vi "ADCP_get_data_packet_list.vi"(8 "error in (no error)":errorcluster, 9 "Node name":string, 10 "Node ID":i32=-1, 11 "ADCP In":refnum<class "ADCP.lvclass">) -> (0 "error out":errorcluster, 1 "Data packets names":string[](array[string]), 2 "Data packets":T2(array[cluster]), 3 "ADCP Out":refnum<class "ADCP.lvclass">)   [LabVIEW 2017, in "ADCP.lvclass"]
uses:
  ADCP.lvclass
  ADCP_Data_Packet_Transmit_Mode.ctl
  ADCP.lvclass/ADCP.ctl
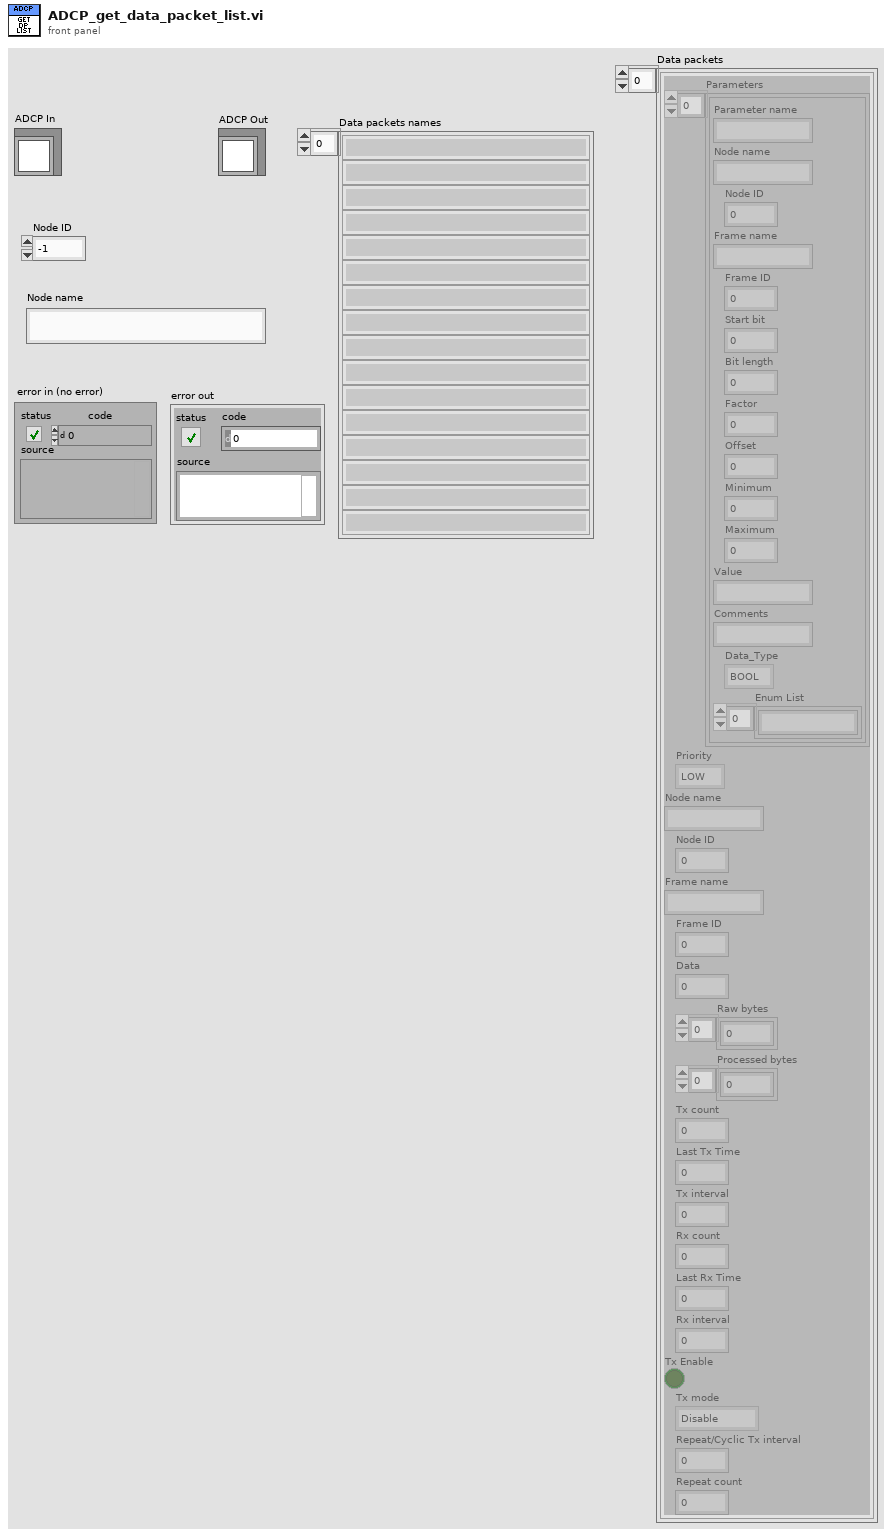
[diagram p1: front panel]
types:
  T1 = typedef "ADCP.lvclass/ADCP_Data_Packet_Transmit_Mode.ctl" = enum16{"Disable", "Single", "Cyclic", "Repeat"}
  T2 = cluster{"Parameters":cluster{"Parameter name":string, "Node name":string, "Node ID":u8, "Frame name":string, "Frame ID":u8, "Start bit":u32, "Bit length":u32, "Factor":dbl, "Offset":dbl, "Minimum":dbl, "Maximum":dbl, "Value":string, "Comments":string, "Data_Type":enum16{"BOOL", "UNSIGNED", "SIGNED", "FLOAT32", "ENUM"}, "Enum List":string[]}[], "Priority":enum16{"LOW", "HIGH"}, "Node name":string, "Node ID":u8, "Frame name":string, "Frame ID":u8, "Data":u32, "Raw bytes":u8[], "Processed bytes":u8[], "Tx count":i32, "Last Tx Time":u32, "Tx interval":u32, "Rx count":i32, "Last Rx Time":u32, "Rx interval":u32, "Tx Enable":bool, "Tx mode":T1, "Repeat/Cyclic Tx interval":u32, "Repeat count":u16}[]
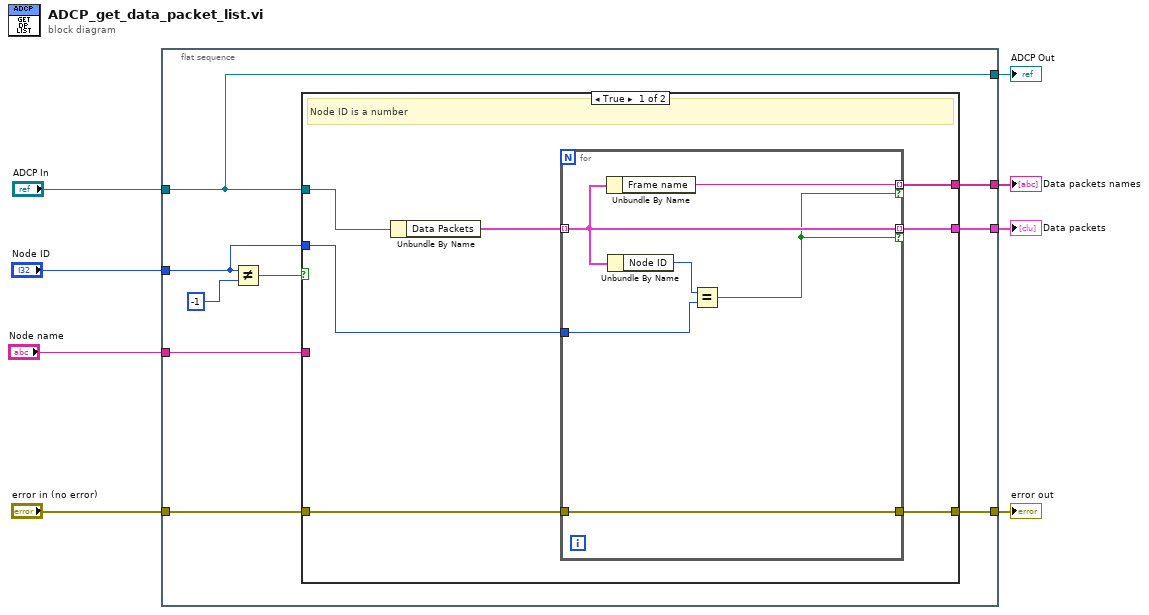
[diagram p0: block diagram]
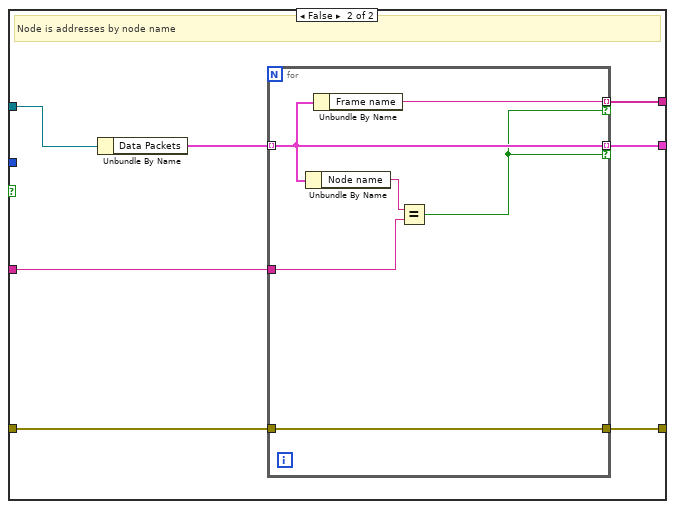
[diagram p2: hidden frame]
diagram:
  n1 = flat-sequence {
    tunnel: "ADCP In" -> [w9]
    tunnel: "Node ID" -> [w12]
    tunnel: "Node name" -> [w13]
    tunnel: "error in (no error)" -> [w15]
    tunnel: [w14] -> w1
    tunnel: [w11] -> w3
    tunnel: [w10] -> w2
    tunnel: [w9] -> w4
    frame #0 {
      n2 = Not Equal?(x=w12, y=-1) -> (x != y?=w16:bool)
      n3 = case shown="True" w16 {
        tunnel: w15 -> [w24 w37]
        tunnel: [w23 w36] -> w14
        tunnel: w13 -> [_ w31]
        tunnel: w9 -> [w22 w35]
        tunnel: w12 -> [w20 _]
        tunnel: [w19 w33] -> w11
        tunnel: [w18 w32] -> w10
        frame True {
          # "Node ID is a number"
          n4 = Unbundle By Name(w22) -> ("Data Packets"=w21:T2)
          n5 = for {
            tunnel: w24 -> [w30]
            tunnel: [w30] -> w23
            tunnel: w21 -> [w26] mode=indexing
            tunnel: w20 -> [w28]
            tunnel: [w27] -> w19 mode=indexing if=w25
            tunnel: [w26] -> w18 mode=indexing if=w25
            n6 = Unbundle By Name(w26) -> ("Frame name"=w27:string)
            n7 = Unbundle By Name(w26) -> ("Node ID"=w29:u8)
            n8 = Equal?(x=w29, y=w28) -> (x = y?=w25:bool)
          }
        }
        frame False {
          # "Node is addresses by node name"
          n9 = Unbundle By Name(w35) -> ("Data Packets"=w34:T2)
          n10 = for {
            tunnel: w37 -> [w43]
            tunnel: [w43] -> w36
            tunnel: w34 -> [w40] mode=indexing
            tunnel: [w41] -> w33 mode=indexing if=w39
            tunnel: [w40] -> w32 mode=indexing if=w39
            tunnel: w31 -> [w38]
            n11 = Unbundle By Name(w40) -> ("Node name"=w42:string)
            n12 = Unbundle By Name(w40) -> ("Frame name"=w41:string)
            n13 = Equal?(x=w42, y=w38) -> (x = y?=w39:bool)
          }
        }
      }
    }
  }
  "ADCP Out" <- w4
  "Data packets names" <- w3
  "Data packets" <- w2
  "error out" <- w1
